vi "MainFrameWork.vi"() -> ()   [LabVIEW 2011]
uses:
  Keypad/Keypad.xctl
  TypeDefs/CTRL to UI Message.ctl
  TypeDefs/CTRL to UI Command.ctl
  TypeDefs/UI to CTRL Message.ctl
  TypeDefs/UI to CTRL Command.ctl
  TypeDefs/User Console Commands.ctl
  TypeDefs/Simulated Database Command.ctl
  TypeDefs/Error Classification.ctl
  TypeDefs/ATM Controller State.ctl
  TypeDefs/UI Items.ctl
panel:
  out "error out":errorcluster
  out "Left Menu 1":string
  out "Left Menu 2":string
  out "Left Menu 3":string
  out "Right Menu 1":string
  out "Right Menu 2":string
  out "Right Menu 3":string
  out "ATM Messages":string
  in  "Left Button 1":bool
  in  "Left Button 2":bool
  in  "Left Button 3":bool
  in  "Right Button 2":bool
  in  "Right Button 3":bool
  in  "Right Button 1":bool
  in  "Keypad":i32(xcontrol)
  in  "Card Slot":bool
  in  "error in (no error)":errorcluster
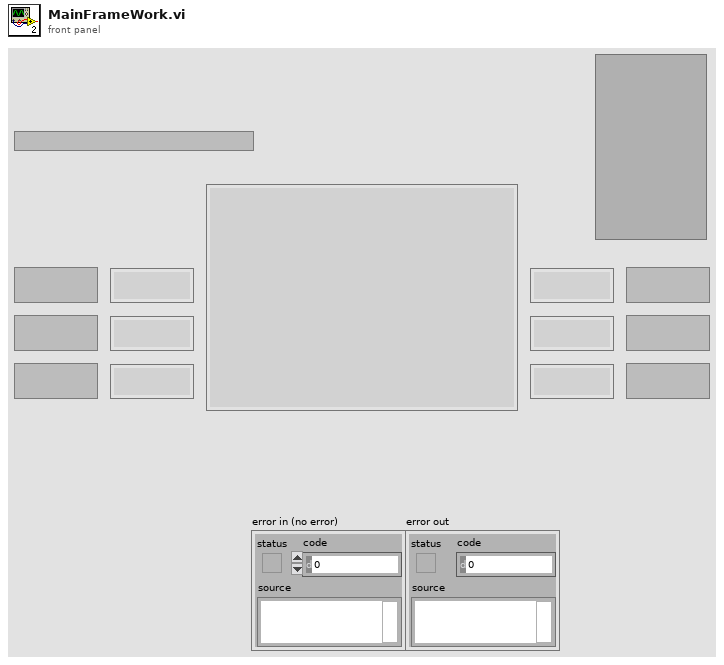
[diagram p1: front panel]
types:
  T1 = enum16{"Init", "Handle", "Check", "Close", "Set Current Account"}
  T2 = typedef "Error Classification.ctl" = enum16{"Minor", "Session", "System"}
  T3 = typedef "Simulated Database Command.ctl" = enum16{"Init", "Look up and Lock Account", "Modify Balance", "Get Record", "Commit Record", "Unlock Record", "Close"}
  T4 = typedef "User Console Commands.ctl" = enum16{"Init", "Set ATM Message", "Set ATM Menus", "Disable Controls", "Wait for Input", "Clear Keypad", "Return Card", "Close"}
  T5 = typedef "UI to CTRL Message.ctl" = cluster{"Command":T6, "Data":variant}
  T6 = typedef "UI to CTRL Command.ctl" = enum16{"Card Inserted", "Keypad Entry", "Button Pressed"}
  T7 = typedef "CTRL to UI Message.ctl" = cluster{"Command":T8, "Data":variant}
  T8 = typedef "CTRL to UI Command.ctl" = enum16{"Display Message", "Return Card", "Stop", "Set Menu", "Clear Keypad", "Disable UI Elements"}
  T9 = typedef "ATM Controller State.ctl" = enum16{"Initial", "Login", "Main Menu", "Balance Inquiry", "Deposit", "Deposit Complete", "Withdrawal", "Withdrawal Success", "Withdrawal Failure", "Terminate", "Lock Out"}
  T10 = typedef "UI Items.ctl" = cluster{"Keypad":bool, "Card Slot":bool, "Left Buttons":bool, "Right Buttons":bool, "ATM Message":bool, "Left Menu":bool, "Right Menu":bool}
  T11 = typedef "Record.ctl" = cluster{"Account Number":u32, "First Name":string, "Last Name":string, "Balance":dbl, "Locked":bool}
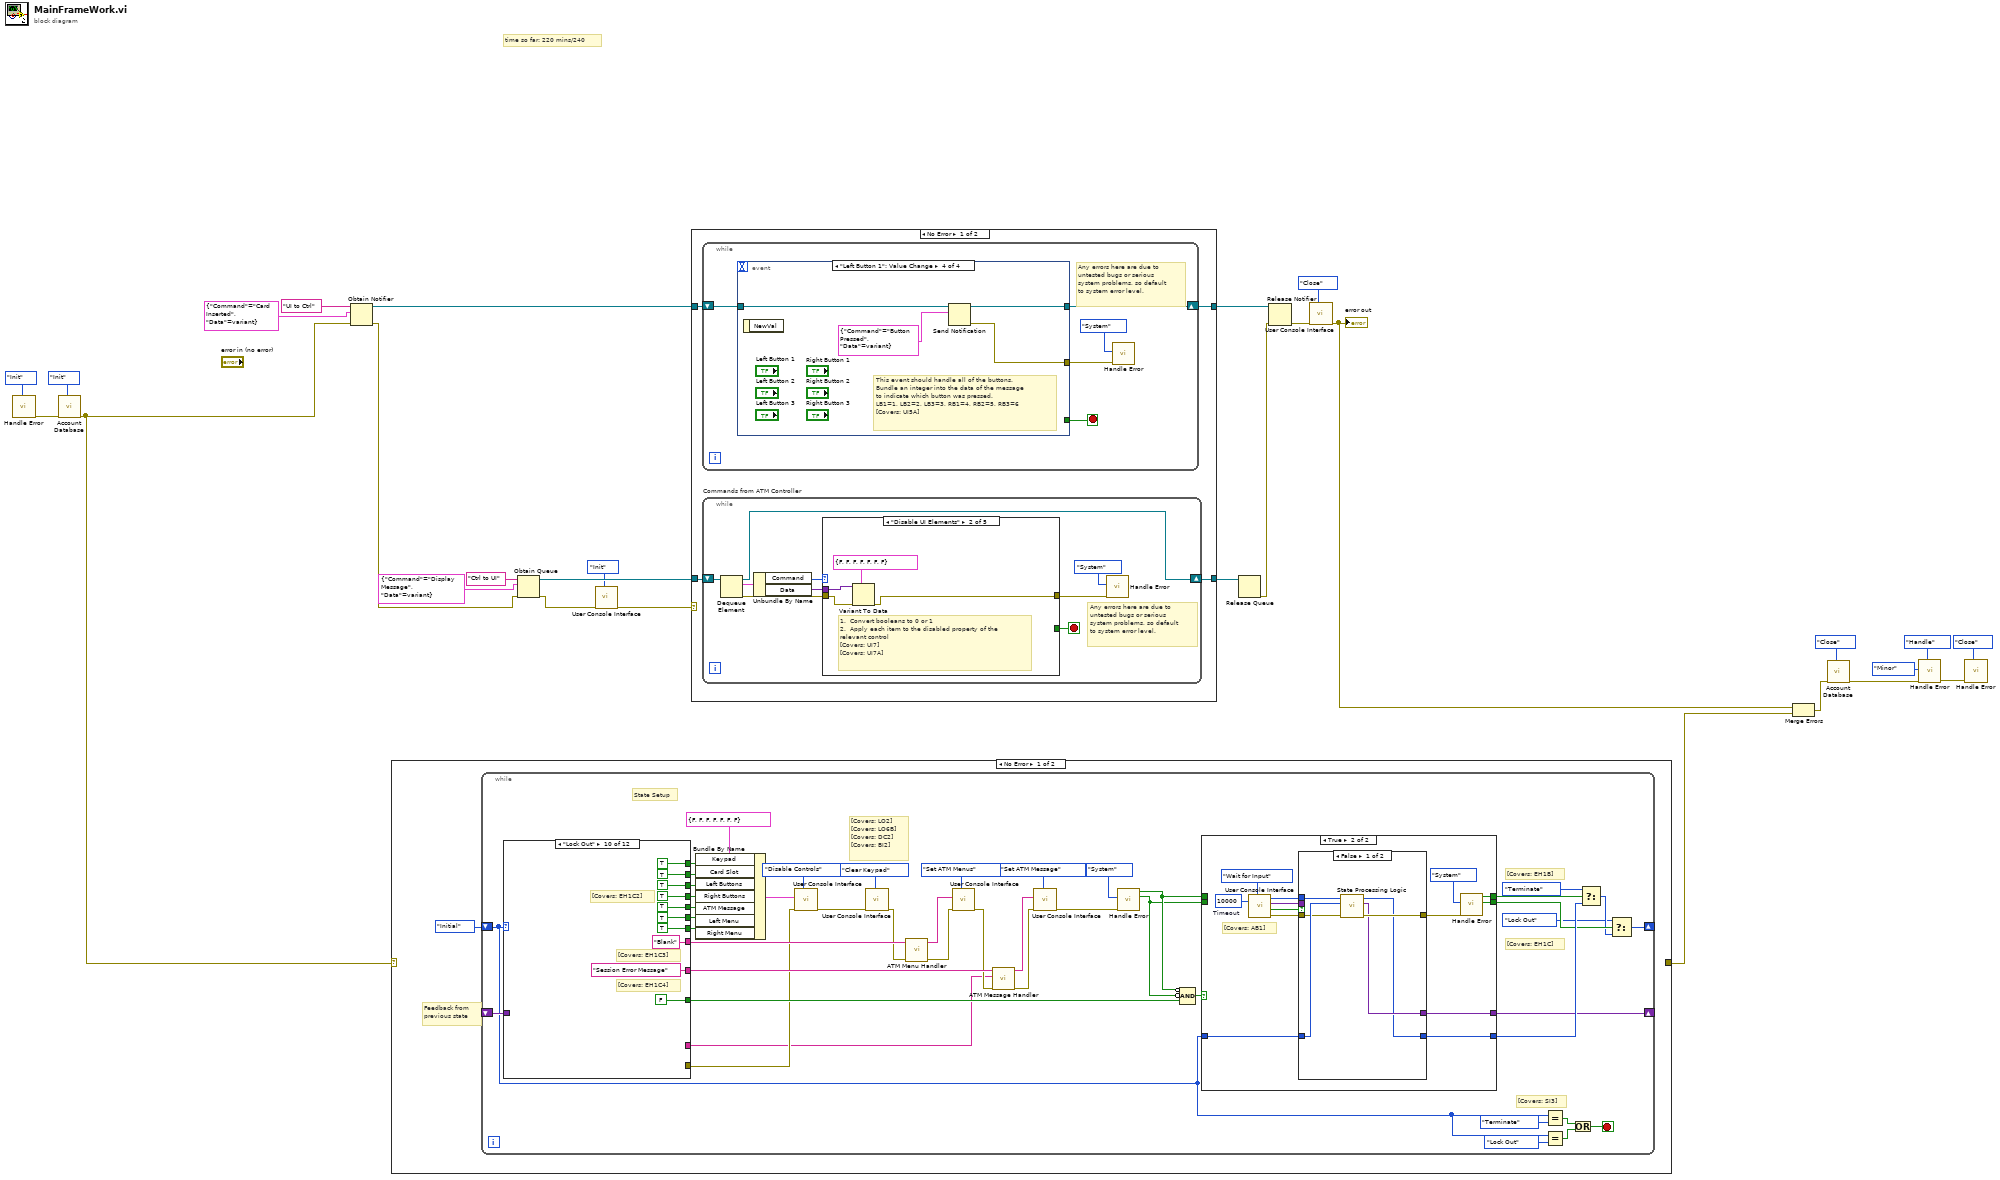
[diagram p0: block diagram]
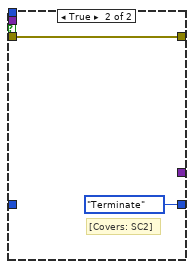
[diagram p3: hidden frame]
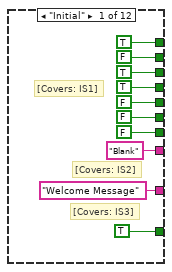
[diagram p4: hidden frame]
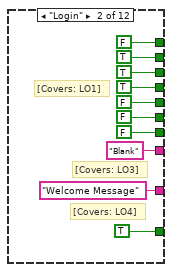
[diagram p5: hidden frame]
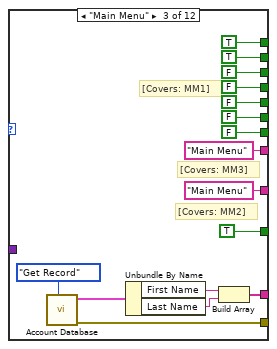
[diagram p6: hidden frame]
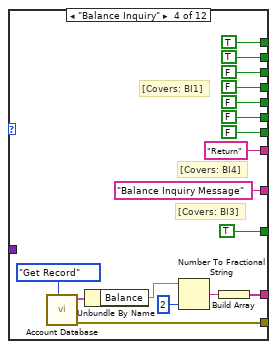
[diagram p7: hidden frame]
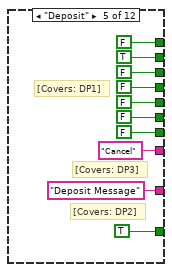
[diagram p8: hidden frame]
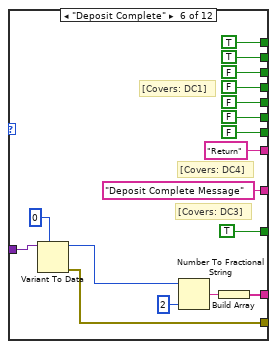
[diagram p9: hidden frame]
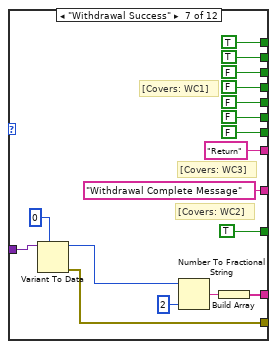
[diagram p10: hidden frame]
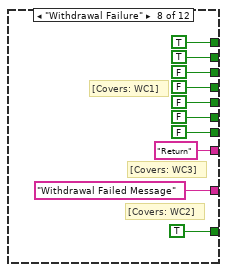
[diagram p11: hidden frame]
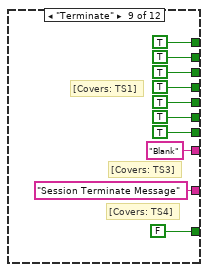
[diagram p12: hidden frame]
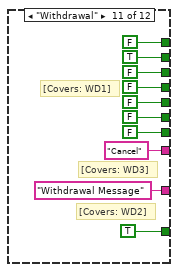
[diagram p13: hidden frame]
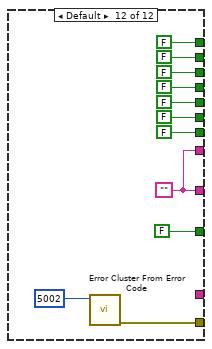
[diagram p14: hidden frame]
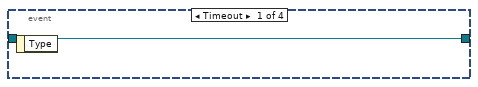
[diagram p16: hidden frame]
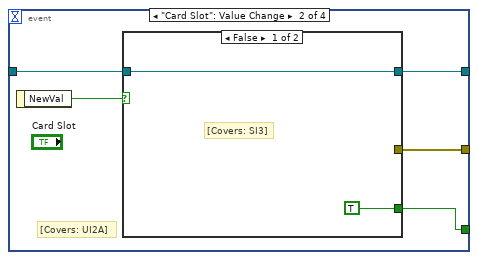
[diagram p17: hidden frame]
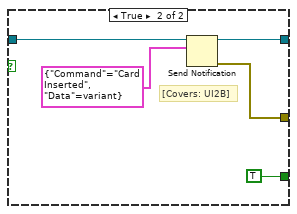
[diagram p18: hidden frame]
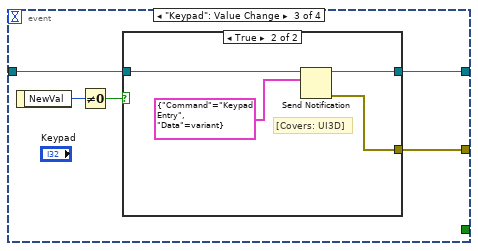
[diagram p19: hidden frame]
diagram:
  # "time so far: 220 mins/240"
  n1 = call "Handle Error.vi"("Command"=T1."Init") -> ("error out"=w11:errorcluster)  [unwired: 8 in, 2 out]
  n2 = call "Account Database.vi"("Command"=Simulated_Database_Command."Init", "error in (no error)"=w11) -> ("error out"=w10:errorcluster)  [unwired: 7 in, 2 out]
  n3 = Obtain Notifier(name (unnamed)="UI to Ctrl", notification data type=T5 {"Command"=enum."Card Inserted", "Data"=variant} ("Cluster"), error in (no error)=w10) -> (notifier out=w23:refnum<notifier>, error out=w19:errorcluster)  [unwired: 1 in, 1 out]
  n4 = case shown="No Error" w10 {
    selector: w10 -> [_ w247]
    tunnel: [_ w247] -> w1
    frame No Error {
      # "Feedback from\nprevious state"
      n5 = while {
        shift-right: [w50] -> _
        shift-left: ATM_Controller_State."Initial" ("State") -> [w30]
        shift-right: [w37] -> _
        shift-left: _ -> [w36]
        stop <- w31 stop-if-true
        # "[Covers: SI3]"
        # "[Covers: LO2]\n[Covers: LO6B]\n[Covers: DC2]\n[Covers: BI2]"
        # "[Covers: EH1C]"
        # "[Covers: EH1B]"
        # "State Setup"
        n6 = case shown="\"Lock Out\"" w30 {
          tunnel: [TRUE ("Keypad") FALSE ("Keypad") TRUE ("Keypad") TRUE ("Keypad") FALSE ("Keypad") TRUE ("Keypad") TRUE ("Keypad") TRUE ("Keypad") TRUE ("Keypad") TRUE ("Keypad") FALSE ("Keypad") FALSE ("Keypad")] -> w73
          tunnel: [FALSE ("Keypad") TRUE ("Keypad") TRUE ("Keypad") TRUE ("Keypad") TRUE ("Keypad") TRUE ("Keypad") TRUE ("Keypad") TRUE ("Keypad") TRUE ("Keypad") TRUE ("Keypad") TRUE ("Keypad") FALSE ("Keypad")] -> w72
          tunnel: [TRUE ("Keypad") TRUE ("Keypad") FALSE ("Keypad") FALSE ("Keypad") FALSE ("Keypad") FALSE ("Keypad") FALSE ("Keypad") FALSE ("Keypad") TRUE ("Keypad") TRUE ("Keypad") FALSE ("Keypad") FALSE ("Keypad")] -> w71
          tunnel: [TRUE ("Keypad") TRUE ("Keypad") FALSE ("Keypad") FALSE ("Keypad") FALSE ("Keypad") FALSE ("Keypad") FALSE ("Keypad") FALSE ("Keypad") TRUE ("Keypad") TRUE ("Keypad") FALSE ("Keypad") FALSE ("Keypad")] -> w70
          tunnel: [FALSE ("Keypad") FALSE ("Keypad") FALSE ("Keypad") FALSE ("Keypad") FALSE ("Keypad") FALSE ("Keypad") FALSE ("Keypad") FALSE ("Keypad") TRUE ("Keypad") TRUE ("Keypad") FALSE ("Keypad") FALSE ("Keypad")] -> w69
          tunnel: [FALSE ("Keypad") FALSE ("Keypad") FALSE ("Keypad") FALSE ("Keypad") FALSE ("Keypad") FALSE ("Keypad") FALSE ("Keypad") FALSE ("Keypad") TRUE ("Keypad") TRUE ("Keypad") FALSE ("Keypad") FALSE ("Keypad")] -> w68
          tunnel: [FALSE ("Keypad") FALSE ("Keypad") FALSE ("Keypad") FALSE ("Keypad") FALSE ("Keypad") FALSE ("Keypad") FALSE ("Keypad") FALSE ("Keypad") TRUE ("Keypad") TRUE ("Keypad") FALSE ("Keypad") FALSE ("Keypad")] -> w67
          tunnel: ["Blank" "Blank" "Main Menu" "Return" "Cancel" "Return" "Return" "Return" "Blank" "Blank" "Cancel" w238] -> w61
          tunnel: ["Welcome Message" "Welcome Message" "Main Menu" "Balance Inquiry Message" "Deposit Message" "Deposit Complete Message" "Withdrawal Complete Message" "Withdrawal Failed Message" "Session Terminate Message" "Session Error Message" "Withdrawal Message" w238] -> w64
          tunnel: [TRUE TRUE TRUE TRUE TRUE TRUE TRUE TRUE FALSE FALSE TRUE FALSE] -> w57
          tunnel: [_ _ w123 w140 _ w164 w181 _ _ _ _ w236] -> w39
          tunnel: [_ _ w119 w138 _ w168 w185 _ _ _ _ _] -> w38
          tunnel: w36 -> [_ _ _ _ _ w165 w182 _ _ _ _ _]
          frame "Initial" {
            # "[Covers: IS3]"
            # "[Covers: IS2]"
            # "[Covers: IS1]"
          }
          frame "Login" {
            # "[Covers: LO4]"
            # "[Covers: LO3]"
            # "[Covers: LO1]"
          }
          frame "Main Menu" {
            # "[Covers: MM2]"
            # "[Covers: MM3]"
            # "[Covers: MM1]"
            n7 = call "Account Database.vi"("Command"=Simulated_Database_Command."Get Record") -> ("error out"=w123:errorcluster, "Record"=w122:T11)  [unwired: 8 in, 1 out]
            n8 = Unbundle By Name(w122) -> ("First Name"=w121:string, "Last Name"=w120:string)
            n9 = Build Array(w121, w120) -> (w119:string[])
          }
          frame "Balance Inquiry" {
            # "[Covers: BI3]"
            # "[Covers: BI4]"
            # "[Covers: BI1]"
            n10 = call "Account Database.vi"("Command"=Simulated_Database_Command."Get Record") -> ("error out"=w140:errorcluster, "Record"=w139:T11)  [unwired: 8 in, 1 out]
            n11 = Unbundle By Name(w139) -> ("Balance"=w136:dbl)
            n12 = Number To Fractional String(number=w136, precision (6)=i16 2) -> (F-format string=w137:string)  [unwired: 2 in]
            n13 = Build Array(w137) -> (w138:string[])
          }
          frame "Deposit" {
            # "[Covers: DP2]"
            # "[Covers: DP3]"
            # "[Covers: DP1]"
          }
          frame "Deposit Complete" {
            # "[Covers: DC3]"
            # "[Covers: DC4]"
            # "[Covers: DC1]"
            n14 = Variant To Data(type=0, Variant=w165) -> (data=w162:i32, error out=w164:errorcluster)  [unwired: 1 in]
            n15 = Number To Fractional String(number=w162, precision (6)=i16 2) -> (F-format string=w167:string)  [unwired: 2 in]
            n16 = Build Array(w167) -> (w168:string[])
          }
          frame "Withdrawal Success" {
            # "[Covers: WC2]"
            # "[Covers: WC3]"
            # "[Covers: WC1]"
            n17 = Variant To Data(type=0, Variant=w182) -> (data=w179:i32, error out=w181:errorcluster)  [unwired: 1 in]
            n18 = Number To Fractional String(number=w179, precision (6)=i16 2) -> (F-format string=w184:string)  [unwired: 2 in]
            n19 = Build Array(w184) -> (w185:string[])
          }
          frame "Withdrawal Failure" {
            # "[Covers: WC2]"
            # "[Covers: WC3]"
            # "[Covers: WC1]"
          }
          frame "Terminate" {
            # "[Covers: TS4]"
            # "[Covers: TS3]"
            # "[Covers: TS1]"
          }
          frame "Lock Out" {
            # "[Covers: EH1C4]"
            # "[Covers: EH1C3]"
            # "[Covers: EH1C2]"
          }
          frame "Withdrawal" {
            # "[Covers: WD2]"
            # "[Covers: WD3]"
            # "[Covers: WD1]"
          }
          frame Default {
            w238 = "" ("Empty String Constant")
            n20 = call <vilib>:"Error Cluster From Error Code.vi"("error code (0)"=5002) -> ("error out"=w236:errorcluster)  [unwired: 8 in]
          }
        }
        n21 = Bundle By Name(cluster=T10 {"Keypad"=FALSE, "Card Slot"=FALSE, "Left Buttons"=FALSE, "Right Buttons"=FALSE, "ATM Message"=FALSE, "Left Menu"=FALSE, "Right Menu"=FALSE} ("UI Items"), "Keypad"=w73, "Card Slot"=w72, "Left Buttons"=w71, "Right Buttons"=w70, "ATM Message"=w69, "Left Menu"=w68, "Right Menu"=w67) -> (w45:T10)
        n22 = call "User Console Interface.vi"("Command"=User_Console_Commands."Disable Controls", "error in (no error)"=w39, "Parameter"=w45) -> ("error out"=w41:errorcluster)  [unwired: 5 in, 3 out]
        n23 = call "User Console Interface.vi"("Command"=User_Console_Commands."Clear Keypad", "error in (no error)"=w41) -> ("error out"=w40:errorcluster)  [unwired: 6 in, 3 out]
        n24 = call "ATM Menu Handler.vi"("error in (no error)"=w40, "Menu State"=w61) -> ("error out"=w60:errorcluster, "Menu Items"=w46:string[])  [unwired: 8 in]
        n25 = call "User Console Interface.vi"("Command"=User_Console_Commands."Set ATM Menus", "error in (no error)"=w60, "Parameter"=w46) -> ("error out"=w63:errorcluster)  [unwired: 5 in, 3 out]
        n26 = call "ATM Message Handler.vi"("error in (no error)"=w63, "Parameters"=w38, "Message Name"=w64) -> ("error out"=w62:errorcluster, "Message"=w47:string)  [unwired: 7 in]
        n27 = call "User Console Interface.vi"("Command"=User_Console_Commands."Set ATM Message", "error in (no error)"=w62, "Parameter"=w47) -> ("error out"=w59:errorcluster)  [unwired: 5 in, 3 out]
        n28 = call "Handle Error.vi"("error in (no error)"=w59, "Classification"=Error_Classification."System") -> ("System Error"=w55:bool, "Session Error"=w56:bool)  [unwired: 7 in, 1 out]
        n29 = Compound Arithmetic op=AND(invert w56, invert w55, w57) -> (w58:bool)
        n30 = case shown="True" w58 {
          tunnel: w56 -> [w77 _]
          tunnel: [w77 w82] -> w54
          tunnel: w55 -> [w76 _]
          tunnel: [w76 w81] -> w52
          tunnel: w30 -> [w75 w79]
          tunnel: [w75 w84] -> w53
          tunnel: [_ w78] -> w37
          frame False {
          }
          frame True {
            w89 = 10000  # Timeout
            # "[Covers: AB1]"
            n31 = call "User Console Interface.vi"("Command"=User_Console_Commands."Wait for Input", "Parameter"=w89) -> ("error out"=w86:errorcluster, "timed out?"=w88:bool, "Parameter Out"=w85:variant, "User Input"=w87:T6)  [unwired: 6 in]
            n32 = case shown="False" w88 {
              tunnel: w87 -> [w95 _]
              tunnel: w86 -> [w94 w97]
              tunnel: w85 -> [_ _]
              tunnel: [w91 ATM_Controller_State."Terminate" ("State")] -> w84
              tunnel: [w93 w97] -> w80
              tunnel: w79 -> [w96 _]
              tunnel: [w92 _] -> w78
              frame False {
                n33 = call "State Processing Logic.vi"("error in"=w94, "Parameter"=w96, "User Input"=w95) -> ("error out"=w93:errorcluster, "Feedback"=w92:variant, "State Out"=w91:T9)  [unwired: 6 in]
              }
              frame True {
                # "[Covers: SC2]"
              }
            }
            n34 = call "Handle Error.vi"("error in (no error)"=w80, "Classification"=Error_Classification."System") -> ("System Error"=w81:bool, "Session Error"=w82:bool)  [unwired: 7 in, 1 out]
          }
        }
        n35 = Equal?(x=w30, y=ATM_Controller_State."Terminate") -> (x = y?=w32:bool)
        n36 = Equal?(x=w30, y=ATM_Controller_State."Lock Out") -> (x = y?=w33:bool)
        n37 = Or(x=w32, y=w33) -> (x .or. y?=w31:bool)
        n38 = Select(t=ATM_Controller_State."Terminate", s=w54, f=w53) -> (s? t:f=w51:T9)
        n39 = Select(t=ATM_Controller_State."Lock Out", s=w52, f=w51) -> (s? t:f=w50:T9)
      }
    }
    frame Error {
    }
  }
  n40 = Obtain Queue(name (unnamed)="Ctrl to UI", element data type=T7 {"Command"=enum."Display Message", "Data"=variant} ("Cluster"), error in (no error)=w19) -> (queue out=w26:refnum<queue>, error out=w18:errorcluster)  [unwired: 2 in, 1 out]
  n41 = call "User Console Interface.vi"("Command"=User_Console_Commands."Init", "error in (no error)"=w18) -> ("error out"=w17:errorcluster)  [unwired: 6 in, 3 out]
  n42 = case shown="No Error" w17 {
    selector: w17 -> [_ w315]
    tunnel: w26 -> [w251 w313]
    tunnel: w23 -> [w250 w314]
    tunnel: [w249 w314] -> w21
    tunnel: [w248 w313] -> w22
    frame No Error {
      n43 = while {
        shift-right: [w252] -> w249
        shift-left: w250 -> [w255]
        stop <- w256 stop-if-true
        # "Any errors here are due to\nuntested bugs or serious\nsystem problems, so default\nto system error level."
        n44 = event shown="[3] \"Left Button 1\": Value Change" {
          selector: _ -> [_ _ _ _]
          dyn-events: _ -> [_ _ _ _]
          timeout: _ -> [_ _ _ _]
          tunnel: [_ w258 _ _] -> w256
          tunnel: w255 -> [w257 w262 w274 w283]
          tunnel: [_ w260 w273 w282] -> w253
          tunnel: [w257 w259 w272 w281] -> w252
          event Timeout {
            n45 = event-data() -> ()  [unwired: 1 in, 1 out]
          }
          event "Card Slot": Value Change {
            # "[Covers: UI2A]"
            n46 = event-data() -> ("NewVal"=w261:bool)  [unwired: 1 in]
            n47 = case shown="False" w261 {
              tunnel: w262 -> [w264 w269]
              tunnel: [_ w267] -> w260
              tunnel: [w264 w266] -> w259
              tunnel: [TRUE ("Stop") TRUE ("Stop")] -> w258
              frame False {
                # "[Covers: SI3]"
              }
              frame True {
                # "[Covers: UI2B]"
                n48 = Send Notification(notification=T5 {"Command"=enum."Card Inserted", "Data"=variant}, notifier=w269) -> (notifier out=w266:refnum<notifier>, error out=w267:errorcluster)  [unwired: 1 in]
              }
            }
          }
          event "Keypad": Value Change {
            n49 = event-data() -> ("NewVal"=w271:i32)  [unwired: 1 in]
            n50 = Not Equal To 0?(x=w271) -> (x != 0?=w270:bool)
            n51 = case shown="True" w270 {
              tunnel: w274 -> [w275 w279]
              tunnel: [_ w277] -> w273
              tunnel: [w275 w276] -> w272
              frame False {
                # "Ignoring zero values prevents messages when\nclearing the keypad and also prevents the user\nfrom entering 0 for a deposit or withdrawal as\nthe reaction to that situation isn't defined by\nthe requirements."
              }
              frame True {
                # "[Covers: UI3D]"
                n52 = Send Notification(notification=T5 {"Command"=enum."Keypad Entry", "Data"=variant}, notifier=w279) -> (notifier out=w276:refnum<notifier>, error out=w277:errorcluster)  [unwired: 1 in]
              }
            }
          }
          event "Left Button 1": Value Change {
            # "This event should handle all of the buttons.\nBundle an integer into the data of the message \nto indicate which button was pressed.\nLB1=1, LB2=2, LB3=3, RB1=4, RB2=5, RB3=6\n[Covers: UI5A]"
            n53 = event-data() -> ()  [unwired: 1 in, 1 out]
            n54 = Send Notification(notification=T5 {"Command"=enum."Button Pressed", "Data"=variant}, notifier=w283) -> (notifier out=w281:refnum<notifier>, error out=w282:errorcluster)  [unwired: 1 in]
          }
        }
        n55 = call "Handle Error.vi"("error in (no error)"=w253, "Classification"=Error_Classification."System") -> ()  [unwired: 7 in, 3 out]
      }
      n56 = while "Commands from ATM Controller" {
        shift-right: [w284] -> w248
        shift-left: w251 -> [w292]
        stop <- w288 stop-if-true
        # "Any errors here are due to\nuntested bugs or serious\nsystem problems, so default\nto system error level."
        n57 = Dequeue Element(queue=w292) -> (queue out=w284:refnum<queue>, element=w291:T7, error out=w287:errorcluster)  [unwired: 2 in, 1 out]
        n58 = Unbundle By Name(w291) -> ("Command"=w290:T8, "Data"=w289:variant)
        n59 = case shown="\"Disable UI Elements\"" w290 {
          tunnel: w289 -> [w296 w300 _ w310 _]
          tunnel: [_ _ TRUE _ _] -> w288
          tunnel: w287 -> [w295 w299 w303 w308 w312]
          tunnel: [w293 w297 w302 w305 w311] -> w286
          frame "Display Message", Default {
            # "[Covers: UI4A]\n[Covers: UI4B]"
            n60 = Variant To Data(error in=w295, Variant=w296) -> (data=→"ATM Messages":string, error out=w293:errorcluster)  [unwired: 1 in]
          }
          frame "Disable UI Elements" {
            # "1.  Convert booleans to 0 or 1\n2.  Apply each item to the disabled property of the\nrelevant control\n[Covers: UI7]\n[Covers: UI7A]"
            n61 = Variant To Data(error in=w299, type=T10 {"Keypad"=FALSE, "Card Slot"=FALSE, "Left Buttons"=FALSE, "Right Buttons"=FALSE, "ATM Message"=FALSE, "Left Menu"=FALSE, "Right Menu"=FALSE} ("UI Items"), Variant=w300) -> (error out=w297:errorcluster)  [unwired: 1 out]
          }
          frame "Return Card" {
            # "[Covers: SI3]"
            n62 = property on="Card Slot" class="Bool (strict)"(error in=w303, "Val(Sgnl)"=FALSE ("Value (Signaling)")) -> (error out=w302:errorcluster)  [unwired: 1 in, 1 out]
          }
          frame "Set Menu" {
            # "[Covers: UI6A]"
            n63 = Variant To Data(error in=w308, type=string[] [], Variant=w310) -> (data=w307:string[], error out=w305:errorcluster)
            n64 = Index Array(array=w307) -> (element=→"Left Menu 1" →"Left Menu 2" →"Left Menu 3" →"Right Menu 1" →"Right Menu 2" →"Right Menu 3":string)  [unwired: 1 in]
          }
          frame "Clear Keypad" {
            # "[Covers: UI3C]"
            n65 = invoke on="Keypad" class="Keypad (strict)" method="Keypad Clear"(error in=w312) -> (error out=w311:errorcluster)  [unwired: 2 in, 2 out]
          }
        }
        n66 = call "Handle Error.vi"("error in (no error)"=w286, "Classification"=Error_Classification."System") -> ()  [unwired: 7 in, 3 out]
      }
    }
    frame Error {
      # "Any errors here indicate the\ninability to properly initialize\nthe system, so the system should\nnot start."
      n67 = call "Handle Error.vi"("error in (no error)"=w315, "Classification"=Error_Classification."System") -> ()  [unwired: 7 in, 3 out]
    }
  }
  n68 = Release Queue(queue=w22) -> (error out=w20:errorcluster)  [unwired: 2 in, 2 out]
  n69 = Release Notifier(notifier=w21, error in (no error)=w20) -> (error out=w14:errorcluster)  [unwired: 1 in, 2 out]
  n70 = call "User Console Interface.vi"("Command"=User_Console_Commands."Close", "error in (no error)"=w14) -> ("error out"=w2:errorcluster)  [unwired: 6 in, 3 out]
  "error out" <- w2
  n71 = Merge Errors(w2, w1) -> (w8:errorcluster)
  n72 = call "Account Database.vi"("Command"=Simulated_Database_Command."Close", "error in (no error)"=w8) -> ("error out"=w6:errorcluster)  [unwired: 7 in, 2 out]
  n73 = call "Handle Error.vi"("Command"=T1."Handle", "error in (no error)"=w6, "Classification"=Error_Classification."Minor") -> ("error out"=w3:errorcluster)  [unwired: 6 in, 2 out]
  n74 = call "Handle Error.vi"("Command"=T1."Close", "error in (no error)"=w3) -> ()  [unwired: 7 in, 3 out]
